vi "reset_OSC.vi"(8 "error in (no error)":errorcluster, 11 "VISA resource name":refnum<visa-resource-name>) -> (0 "error out":errorcluster, 3 "VISA resource name out":refnum<visa-resource-name>)   [LabVIEW 2011]
doc: "Establishes communication with the instrument and performs an instrument reset. \n\nThis VI also places the instrument in a default state needed for other instrument driver operations."
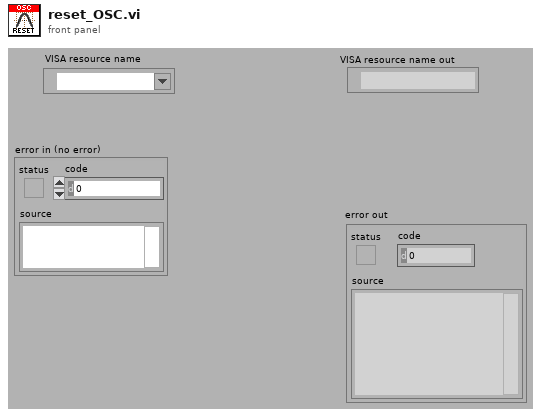
[diagram p1: front panel]
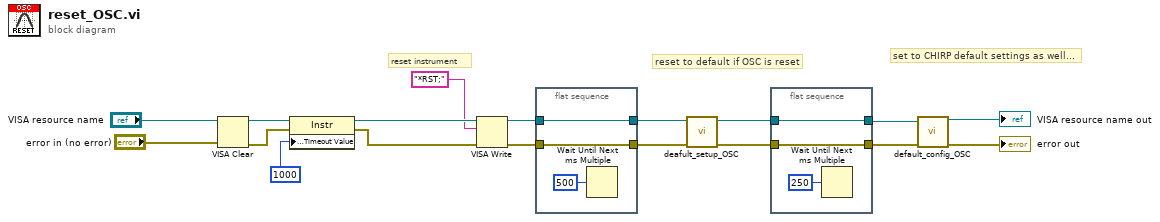
[diagram p0: block diagram]
diagram:
  # "reset instrument"
  # "set to CHIRP default settings as well..."
  # "reset to default if OSC is reset"
  n1 = VISA Clear(VISA resource name="VISA resource name", error in (no error)="error in (no error)") -> (VISA resource name out=w18:refnum<visa-resource-name>, error out=w17:errorcluster)
  n2 = property on="Property Node" class="Instr"(reference=w18, error in=w17, "General Settings:Timeout Value"=u32 1000) -> (reference out=w13:refnum<visa-resource-name>, error out=w12:errorcluster)
  n3 = VISA Write(VISA resource name=w13, write buffer="*RST;", error in (no error)=w12) -> (VISA resource name out=w15:refnum<visa-resource-name>, error out=w14:errorcluster)  [unwired: 1 out]
  n4 = flat-sequence {
    tunnel: w15 -> [w20]
    tunnel: [w20] -> w11
    tunnel: w14 -> [w19]
    tunnel: [w19] -> w10
    frame #0 {
      n5 = Wait Until Next ms Multiple(millisecond multiple=u32 500) -> ()  [unwired: 1 out]
    }
  }
  n6 = call "deafult_setup_OSC.vi"("error in (no error)"=w10, "VISA resource name"=w11) -> ("error out"=w8:errorcluster, "VISA resource name out"=w9:refnum<visa-resource-name>)  [unwired: 8 in]
  n7 = flat-sequence {
    tunnel: w9 -> [w23]
    tunnel: [w23] -> w7
    tunnel: w8 -> [w22]
    tunnel: [w22] -> w6
    frame #0 {
      n8 = Wait Until Next ms Multiple(millisecond multiple=u32 250) -> ()  [unwired: 1 out]
    }
  }
  n9 = call "default_config_OSC.vi"("VISA resource in"=w7, "error in (no error)"=w6) -> ("VISA resource name out"=→"VISA resource name out":refnum<visa-resource-name>, "error out"=→"error out":errorcluster)  [unwired: 12 in]
